vi "Draw Body Index Frame.vi"(8 "Error In":errorcluster, 10 "Byte Array":u8[](array[numeric]), 11 "Image":T1) -> (0 "Error Out":errorcluster, 3 "Image Out":T1)   [LabVIEW 2014, in "LVH-KinectOne.lvlib"]
doc: "Converts the Body Index data to an RGB U32 IMAQ Image."
uses:
  LVH-KinectOne.lvlib
  <vilib>/vision/Image Controls.llb/IMAQ Image.ctl
  Private/Frame Description FGV [Body Index].vi
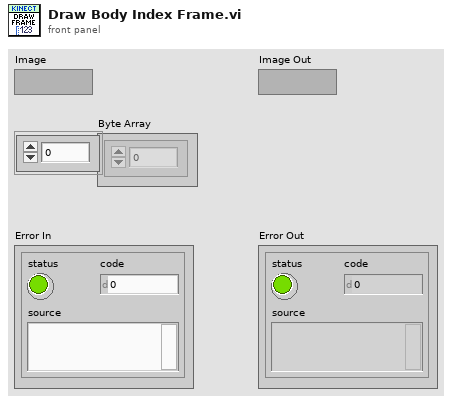
[diagram p1: front panel]
types:
  T1 = typedef "IMAQ Image.ctl" = refnum<image>
  T2 = typedef "LVH-KinectOne.lvlib/FrameDescription.ctl" = cluster{"BytesPerPixel":u32, "DiagonalFieldOfView":sgl, "Height":i32, "HorizontalFieldOfView":sgl, "LengthInPixels":u32, "VerticalFieldOfView":sgl, "Width":i32}
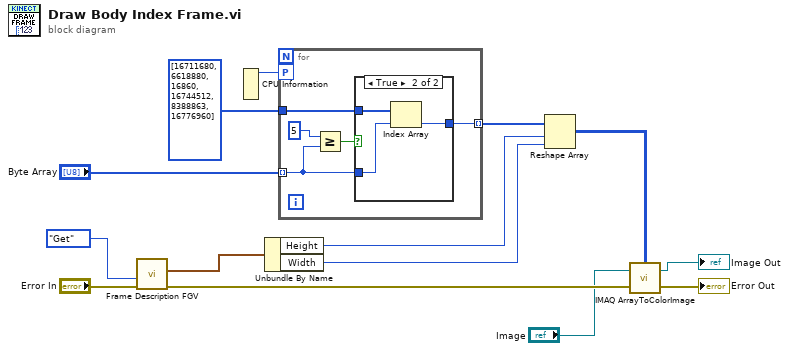
[diagram p0: block diagram]
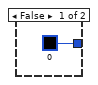
[diagram p2: hidden frame]
diagram:
  n1 = call-poly "Frame Description FGV.vi"("error in (no error)"="Error In", "Command"=enum16{"Get", "Set"}."Get") -> ("error out"=w7:errorcluster, "FrameDescription"=w9:T2)  [unwired: 8 in]
  n2 = CPU Information() -> (4:w13:i32)  [unwired: 3 out]
  n3 = Unbundle By Name(w9) -> ("Height"=w12:i32, "Width"=w11:i32)
  n4 = for {
    tunnel: "Byte Array" -> [w16] mode=indexing
    tunnel: u32[] [16711680, 6618880, 16860, 16744512, 8388863, 16776960] -> [w19]
    tunnel: [w15] -> w10 mode=indexing
    workers-P: w13 -> [_]
    n5 = Greater Or Equal?(x=u8 5, y=w16) -> (x >= y?=w17:bool)
    n6 = case shown="True" w17 {
      tunnel: w19 -> [_ w23]
      tunnel: w16 -> [_ w22]
      tunnel: [u32 0 w21] -> w15
      frame False {
      }
      frame True {
        n7 = Index Array(array=w23, index=w22) -> (element=w21:u32)
      }
    }
  }
  n8 = Reshape Array(w10, w12, w11) -> (w8:u32[][])
  n9 = call "IMAQ ArrayToColorImage"("Image Pixels (U32)"=w8, "Image"="Image", "error in (no error)"=w7) -> ("Image Out"=→"Image Out":T1, "error out"=→"Error Out":errorcluster)  [unwired: 2 in]
